vi "Cargo Ship Score - After Elevator Height.vi"(6 "Synchronization":enum16{"Start", "Wait"}(ring), 7 "Description":string, 8 "Command Info In":T3, 11 "Clear Queue? (F)":bool) -> (0 "Command Info Out":T3)   [LabVIEW 2019]
doc: "This template has a parameter to control whether it waits for the command to complete or not. This is useful for operations that have a timed duration or a sensor-based duration. \n\nBe sure to right-click and select New from Template and save with a new command name."
uses:
  <vilib>/Rock Robotics/WPI/Framework/Command Status Info.ctl
  <vilib>/Rock Robotics/WPI/Framework/Completion Status.ctl
  <vilib>/Rock Robotics/WPI/Framework/Completion Notifier.ctl
  Implementation/Sequencer Type.ctl
  Implementation/All Commands.ctl
  Implementation/Subsystem Sequencer Setpoints.ctl
  Implementation/Subsystem Sequencer Operations.ctl
panel:
  in  "Sequence":T1[](array[typedef])=[{"Cmd"=enum."Wait ms", "Value"=1300.0}, {"Cmd"=enum."Wrist - Set Position", "Value"=55.0}, {"Cmd"=enum."Wait ms", "Value"=200.0}, {"Cmd"=enum."Roller - Set Position", "Value"=0.3}, {"Cmd"=enum."Wait ms", "Value"=1000.0}, {"Cmd"=enum."Roller - Off", "Value"=0.0}, {"Cmd"=enum."Wrist - Up", "Value"=0.0}]
  # "Right click the ARRAY, Data Operation --> Set Current Values as Default"
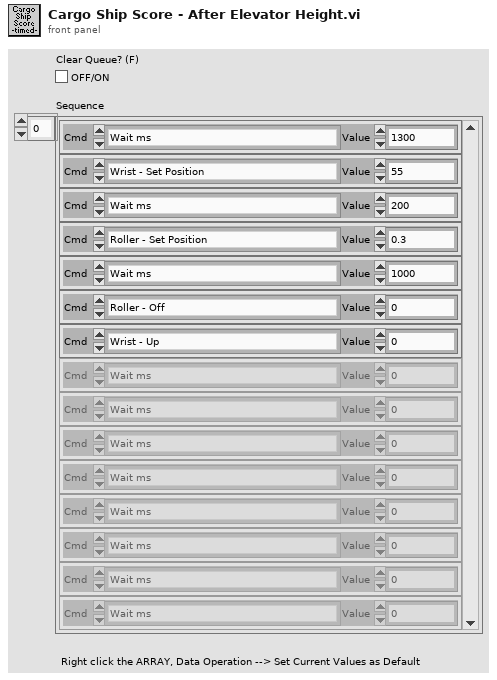
[diagram p1: front panel]
types:
  T1 = typedef "Sequencer Type.ctl" = cluster{"Cmd":T2, "Value":dbl}
  T2 = typedef "All Commands.ctl" = enum16{"Wait ms", "Drive - Stop Driving", "Drive - Drive Distance Straight", "Elevator - Elevator Stop", "Elevator - Elevator Set Position Wait", "Elevator - Elevator Set Position Start", "Elevator - Wait for Down Fast", "Wrist - Up", "Wrist - Down", "Wrist - Set Position", "Beak - Extend", "Beak - Retract", "Beak - Open", "Beak - Close", "Roller - Off", "Roller - Out", "Roller - In", "Roller - Set Position", "Roller - Wait for Cargo", "Drive - Set Power Straight", "Elevator - Wait Until Stopped", "Leg  - Piston Engage", "Wrist - Set Position Override", "Elevator - Wait for Up Fast", "Elevator - Jog", "Elevator - Wait for Position"}
  T3 = typedef "Command Status Info.ctl" = cluster{"Name":string, "Status":T4, "notifier out":T5}
  T4 = typedef "Completion Status.ctl" = enum16{"Successful", "Aborted", "Incomplete"}
  T5 = typedef "Completion Notifier.ctl" = refnum<notifier>
  T6 = typedef "Subsystem Sequencer Setpoints.ctl" = cluster{"Operation":T7, "Setpoint":dbl, "Duration":dbl}
  T7 = typedef "Subsystem Sequencer Operations.ctl" = enum16{"Reserve", "Read Current", "Run Sequence"}
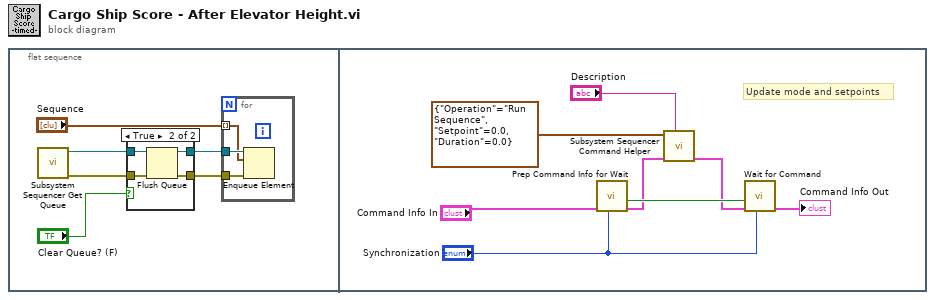
[diagram p0: block diagram]
diagram:
  n1 = flat-sequence {
    frame #0 {
      n2 = call "Subsystem Sequencer Get Queue.vi"() -> ("error out"=w4:errorcluster, "queue out"=w6:refnum<queue>)  [unwired: 10 in]
      n3 = case shown="True" "Clear Queue? (F)" {
        tunnel: w6 -> [w8 w12]
        tunnel: [w8 w11] -> w5
        tunnel: w4 -> [w7 w10]
        tunnel: [w7 w9] -> w3
        frame False {
        }
        frame True {
          n4 = Flush Queue(queue=w12, error in (no error)=w10) -> (queue out=w11:refnum<queue>, error out=w9:errorcluster)  [unwired: 1 out]
        }
      }
      n5 = for {
        tunnel: w5 -> [w15]
        tunnel: w3 -> [w14]
        tunnel: "Sequence" -> [w13] mode=indexing
        n6 = Enqueue Element(queue=w15, element=w13, error in (no error)=w14) -> ()  [unwired: 1 in, 3 out]
      }
    }
    frame #1 {
      # "Update mode and setpoints"
      n7 = call <vilib>:"Prep Command Info for Wait.vi"("Synchronication"="Synchronization", "Command Info"="Command Info In") -> ("Command Info"=w21:T3, "Allocated"=w22:bool)  [unwired: 8 in]
      n8 = call "Subsystem Sequencer Command Helper.vi"("Description"="Description", "Command Info In"=w21, "SubSystem Data"=T6 {"Operation"=enum."Run Sequence", "Setpoint"=0.0, "Duration"=0.0}) -> ("Command Info Out"=w18:T3)  [unwired: 6 in, 2 out]
      n9 = call <vilib>:"Wait for Command.vi"("Synchronication"="Synchronization", "Command Info in"=w18, "Allocated"=w22) -> ("Command Info out"=→"Command Info Out":T3)  [unwired: 8 in]
    }
  }
